vi "TDMS - File Viewer.vi"(4 "error in (no error)":errorcluster, 7 "file path":path) -> (0 "error out":errorcluster, 3 "file path out":path)   [LabVIEW 2020]
doc: "Opens the .tdms file specified in the <B>file in</B> input and presents the file data in the TDMS File Viewer dialog box."
uses:
  <vilib>/Utility/tdmsutil.llb/fileViewerConfigData.ctl
  <vilib>/Utility/error.llb/DialogType.ctl
  <vilib>/event_ctls.llb/sizeaction.ctl
  <vilib>/event_ctls.llb/panelstate.ctl
  <vilib>/Utility/tdmsutil.llb/TDMSFileViewerLocalizedText.vi
  Instance           1 26Saved   TDMS - File Viewer .vi
panel:
  out "LastXScaleFormat":u8
  out "TotalCount":u64
  out "Temp Configuration":T1
  in  "LastTopLeftValue":u64
  out "Resize?":bool
  in  "Help":bool
  in  "Status":string
  in  "Quit":bool
  in  "Settings...":bool
  in  "Properties / Values / Graph":T2(tab)
  in  "Properties":i32(listbox)
  in  "Go To":bool
  in  "Scrollbar":u64(c297)
  in  "Raw data values":i32(listbox)
  out "Waveform Graph":waveform(dbl)[](graph)
  in  "File contents":string(tree)
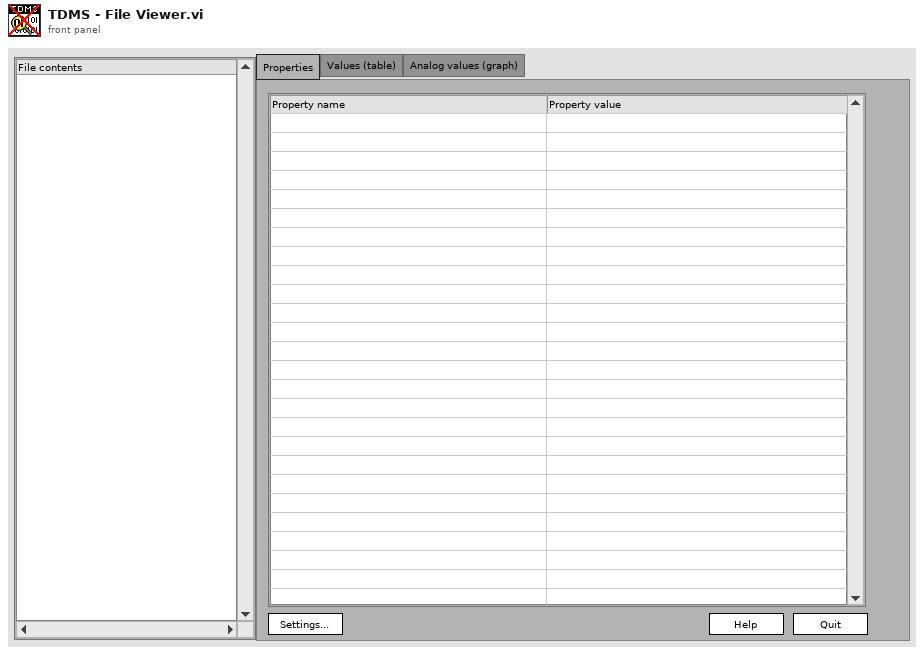
[diagram p1: front panel]
types:
  T1 = typedef "fileViewerConfigData.ctl" = cluster{"Show all (table)":bool, "Show all (graph)":bool, "limit (table)":u64, "limit (graph)":u64, "no show":bool, "start (table)":u64, "start (graph)":u64}
  T2 = enum32{"Properties", "Values (table)", "Analog values (graph)"}
  T3 = enum16{"open", "open or create", "create or replace", "create", "open (read-only)"}
  T4 = cluster{"Tree":refnum<vi>, "Tab Control":refnum<vi>, "property list":refnum<vi>, "raw data list":refnum<vi>, "Waveform Graph":refnum<vi>, "Ok":refnum<vi>, "Ok 2":refnum<vi>, "Ok 3":refnum<vi>, "Ok 4":refnum<vi>, "Scrollbar":refnum<vi>, "Ok 5":refnum<vi>, "TopLeftValue":refnum<vi>, "TotalCount":refnum<vi>}
  T5 = typedef "panelstate.ctl" = enum32{"Standard", "Minimized", "Maximized"}
  T6 = typedef "sizeaction.ctl" = enum32{"Minimized", "Maximized", "Resized"}
  T7 = cluster{"Shift":bool, "Ctrl":bool, "Alt":bool, "Cmd":bool, "Opt":bool}
  T8 = typedef "LVRectTypeDef.ctl" = cluster{"Left":i16, "Top":i16, "Right":i16, "Bottom":i16}
  T9 = typedef "LVRowAndColumnUnsignedTypeDef.ctl" = cluster{"Row":u32, "Column":u32}
  T10 = typedef "DialogType.ctl" = u16
  T11 = typedef "eventvkey.ctl" = enum16{"ASCII", "Enter", "Return", "Shift", "Ctrl", "Alt", "Cmd", "Opt", "Caps", "NumLock", "Clear", "Break", "Up", "Down", "Left", "Right", "Insert", "Delete", "Home", "End", "PageUp", "PageDown", "Escape", "Help", "Pause", "ScrollLock", "F1", "F2", "F3", "F4", "F5", "F6", "F7", "F8", "F9", "F10", "F11", "F12", "F13", "F14", "F15", "F16", "F17", "F18", "F19", "F20", "F21", "F22", "F23", "F24", "Play", "VolumeUp", "VolumeDown", "Mute", "Two Byte Char"}
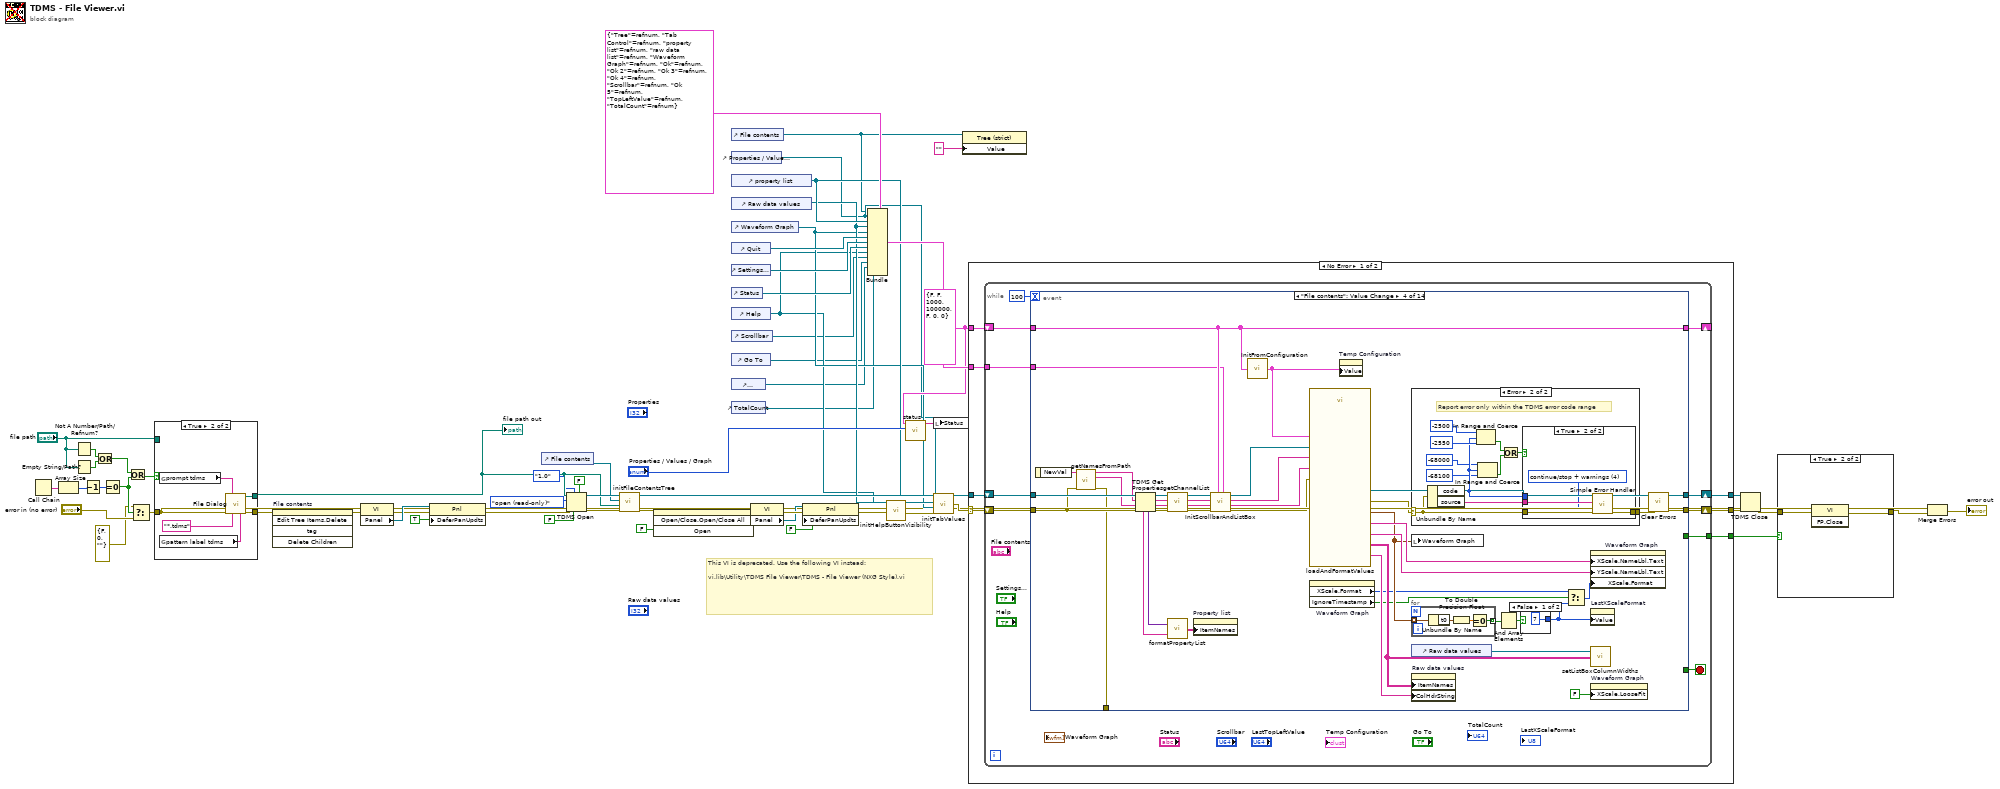
[diagram p0: block diagram]
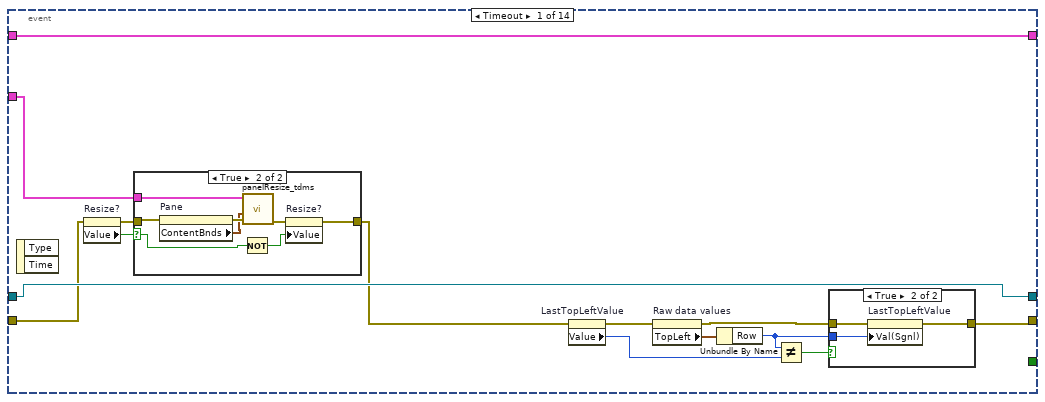
[diagram p3: hidden frame]
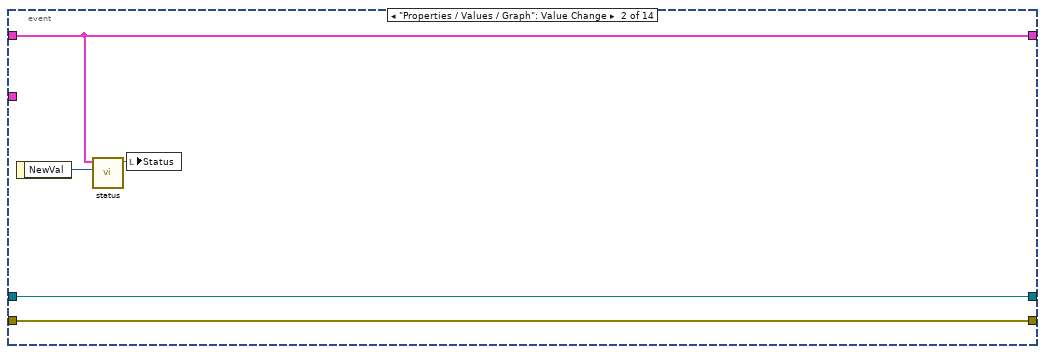
[diagram p6: hidden frame]
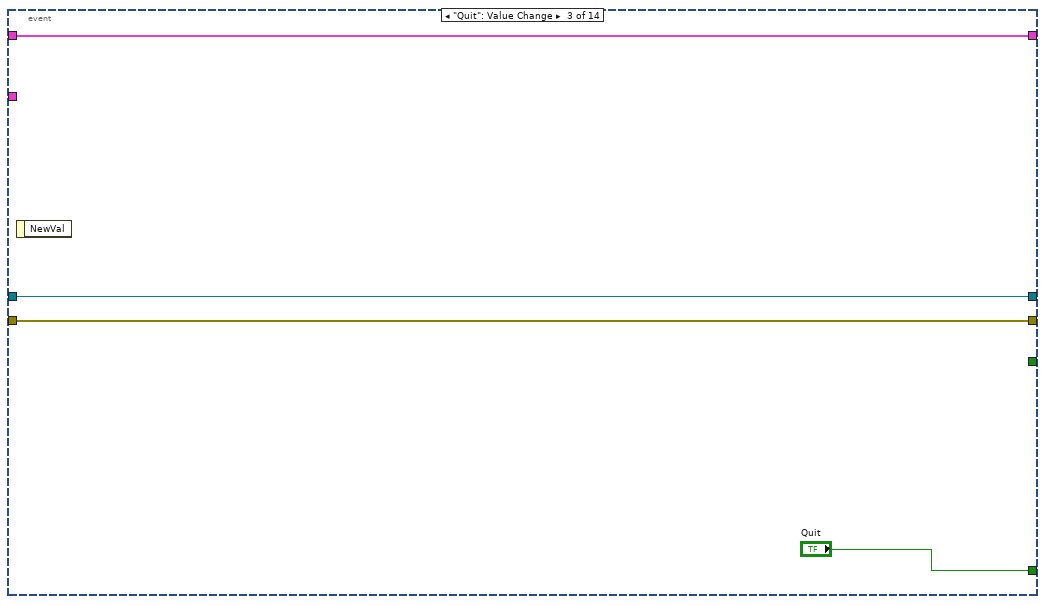
[diagram p7: hidden frame]
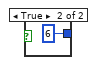
[diagram p8: hidden frame]
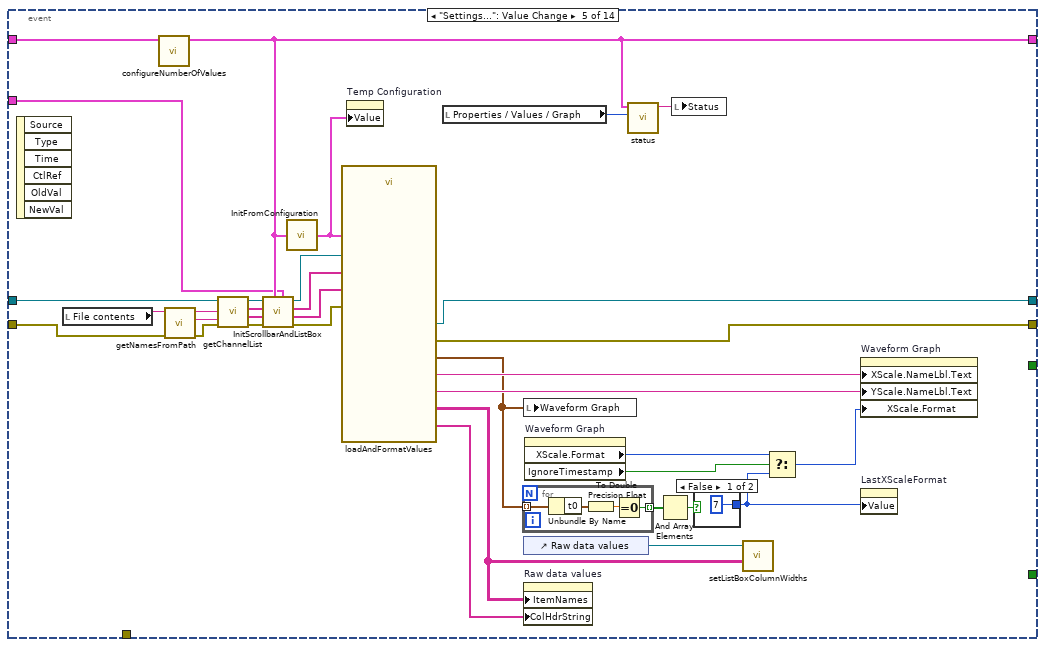
[diagram p11: hidden frame]
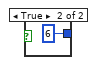
[diagram p12: hidden frame]
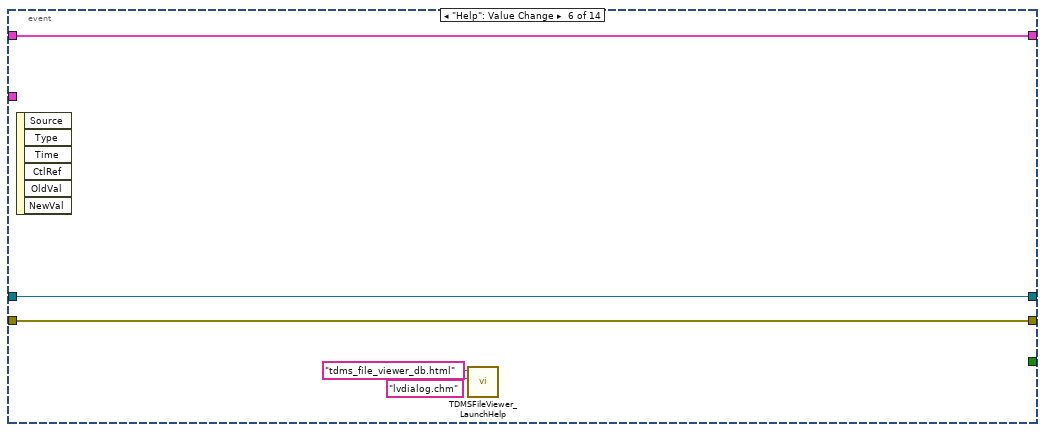
[diagram p13: hidden frame]
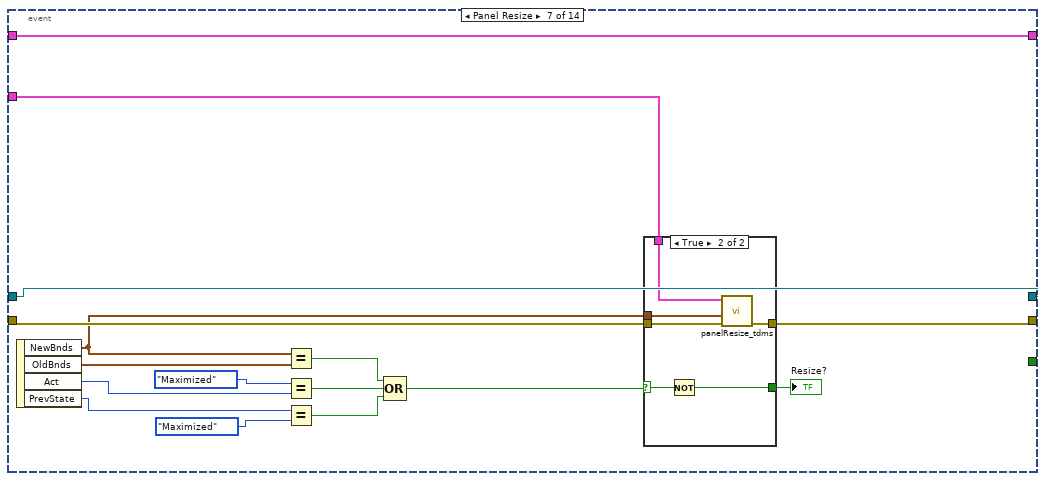
[diagram p14: hidden frame]
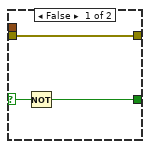
[diagram p15: hidden frame]
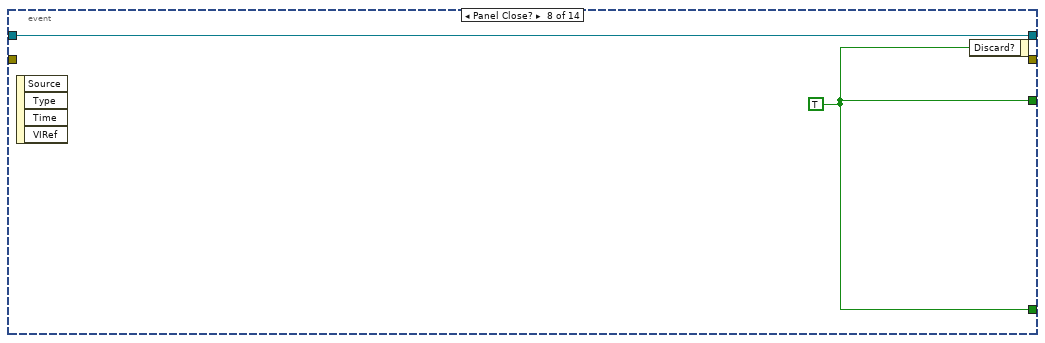
[diagram p16: hidden frame]
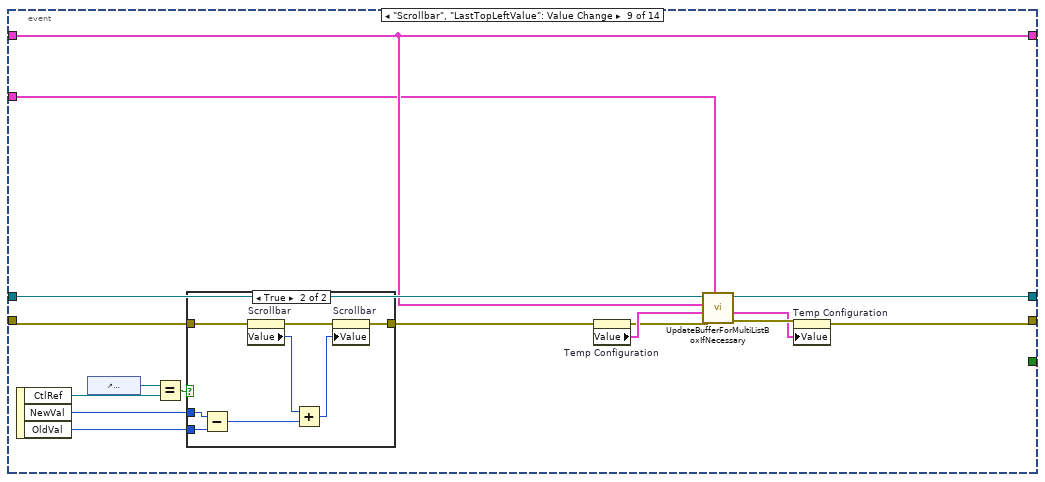
[diagram p17: hidden frame]
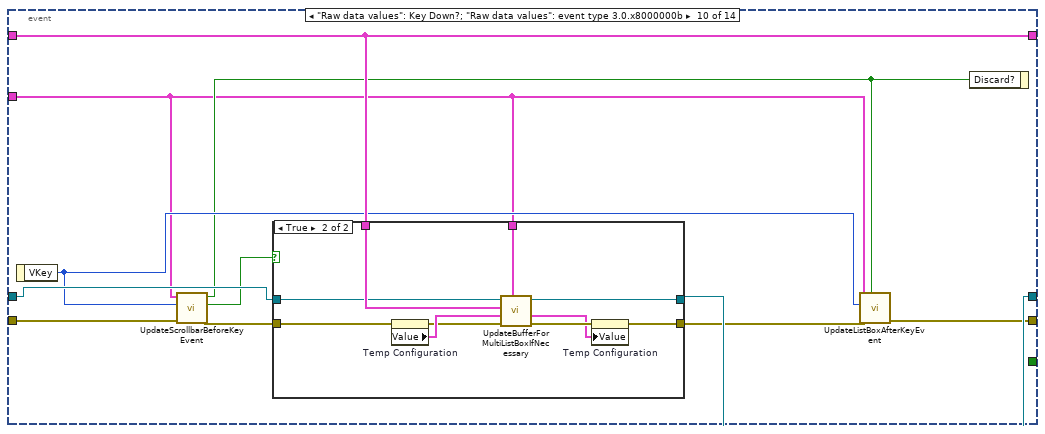
[diagram p19: hidden frame]
diagram:
  w27 = T1 {"Show all (table)"=FALSE, "Show all (graph)"=FALSE, "limit (table)"=1000, "limit (graph)"=100000, "no show"=FALSE, "start (table)"=0, "start (graph)"=0} ("TDMS File Viewer Configuration")
  # "This VI is deprecated. Use the following VI instead:\n\nvi.lib\\Utility\\TDMS File Viewer\\TDMS - File Viewer (NXG Style).vi"
  n1 = Call Chain() -> (call chain=w42:string[])
  n2 = Array Size(array=w42) -> (size(s)=w40:i32)
  n3 = Not A Number/Path/Refnum?(number/path/refnum="file path") -> (NaN/Path/Refnum?=w44:bool)
  n4 = Empty String/Path?(string/path="file path") -> (empty?=w43:bool)
  n5 = Decrement(x=w40) -> (x-1=w39:i32)
  n6 = Or(x=w44, y=w43) -> (x .or. y?=w41:bool)
  n7 = Equal To 0?(x=w39) -> (x = 0?=w25:bool)
  n8 = Or(x=w41, y=w25) -> (x .or. y?=w38:bool)
  n9 = Select(t=errorcluster {"status"=FALSE, "code"=0, "source"=""}, s=w25, f="error in (no error)") -> (s? t:f=w6:errorcluster)
  n10 = case shown="True" w38 {
    tunnel: [w63 w69] -> w31
    tunnel: "file path" -> [w63 _]
    tunnel: [w62 w67] -> w30
    tunnel: w6 -> [w62 w66]
    frame False {
    }
    frame True {
      n11 = global read "TDMSFileViewerLocalizedText.vi" "prompt tdms"() -> (w65:string)
      n12 = global read "TDMSFileViewerLocalizedText.vi" "pattern label tdms"() -> (w64:string)
      n13 = call "File Dialog"("prompt"=w65, "error in"=w66, "pattern (all files)"="*.tdms", "pattern label"=w64) -> ("selected path"=w69:path, "error out"=w67:errorcluster)  [unwired: 3 in, 7 out]
    }
  }
  "file path out" <- w31
  n14 = invoke on="File contents" class="Tree (strict)" method="Edit Tree Items.Delete"(error in=w30) -> (error out=w52:errorcluster)  [unwired: 4 in, 4 out]
  n15 = property class="VI"(error in=w52) -> (error out=w53:errorcluster, "Panel"=w54:refnum<vi>)  [unwired: 1 in, 1 out]
  n16 = property class="Pnl"(reference=w54, error in=w53, "DeferPanUpdts"=TRUE ("Defer Panel Updates")) -> (error out=w56:errorcluster)  [unwired: 1 out]
  n17 = control-ref of="File contents"() -> (w32:refnum<vi>)
  n18 = TDMS Open(5:FALSE ("create index file? (T)"), 6:FALSE ("disable buffering (T)"), 7:enum16{"1.0", "2.0"}."1.0" ("file format version (2.0)"), 8:w56, 10:T3."open (read-only)" ("operation"), 11:w31) -> (0:w61:errorcluster, 3:w60:refnum<k34>)  [unwired: 1 in]
  n19 = call <vilib>:"initFileContentsTree.vi"("error in (no error)"=w61, "file path"=w31, "Tree Refnum"=w32, "tdms file"=w60) -> ("error out"=w48:errorcluster, "tdms file out"=w59:refnum<k34>)  [unwired: 2 out]
  n20 = invoke on="File contents" class="Tree (strict)" method="Open/Close.Open/Close All"(error in=w48, "Open"=FALSE ("Open?")) -> (error out=w47:errorcluster)  [unwired: 2 in, 3 out]
  n21 = control-ref of="File contents"() -> (w13:refnum<vi>)
  n22 = control-ref of="Properties / Values / Graph"() -> (w14:refnum<vi>)
  n23 = control-ref of="property list"() -> (w17:refnum<vi>)
  n24 = control-ref of="Raw data values"() -> (w16:refnum<vi>)
  n25 = control-ref of="Waveform Graph"() -> (w15:refnum<vi>)
  n26 = control-ref of="Quit"() -> (w36:refnum<vi>)
  n27 = control-ref of="Settings..."() -> (w34:refnum<vi>)
  n28 = control-ref of="Status"() -> (w29:refnum<vi>)
  n29 = control-ref of="Help"() -> (w9:refnum<vi>)
  n30 = control-ref of="Scrollbar"() -> (w5:refnum<vi>)
  n31 = control-ref of="Go To"() -> (w4:refnum<vi>)
  n32 = control-ref of="LastTopLeftValue"() -> (w3:refnum<vi>)
  n33 = control-ref of="TotalCount"() -> (w2:refnum<vi>)
  n34 = property class="VI"(error in=w47) -> (error out=w50:errorcluster, "Panel"=w49:refnum<vi>)  [unwired: 1 in, 1 out]
  n35 = property class="Pnl"(reference=w49, error in=w50, "DeferPanUpdts"=FALSE ("Defer Panel Updates")) -> (error out=w11:errorcluster)  [unwired: 1 out]
  n36 = Bundle(cluster=T4 {"Tree"=refnum, "Tab Control"=refnum, "property list"=refnum, "raw data list"=refnum, "Waveform Graph"=refnum, "Ok"=refnum, "Ok 2"=refnum, "Ok 3"=refnum, "Ok 4"=refnum, "Scrollbar"=refnum, "Ok 5"=refnum, "TopLeftValue"=refnum, "TotalCount"=refnum} ("control refs"), "Tree"=w13, "Tab Control"=w14, "property list"=w17, "raw data list"=w16, "Waveform Graph"=w15, "Ok"=w36, "Ok 2"=w34, "Ok 3"=w29, "Ok 4"=w9, "Scrollbar"=w5, "Ok 5"=w4, "TopLeftValue"=w3, "TotalCount"=w2) -> (w37:T4)
  n37 = call <vilib>:"initHelpButtonVisibility.vi"("error in"=w11, "Help"=w9) -> ("error out"=w10:errorcluster)  [unwired: 9 in]
  n38 = call <vilib>:"status.vi"("tab sheet"="Properties / Values / Graph", "TDMS File Viewer Configuration"=w27) -> ("status"=w28:string)  [unwired: 5 out]
  n39 = local write "Status"(w28) -> ()
  n40 = call <vilib>:"initTabValues.vi"("properties"=w17, "Values"=w16, "waveform"=w15, "error in"=w10, "Properties / Values / Graph"=w14) -> ("error out"=w18:errorcluster)
  n41 = property class="Tree (strict)"(reference=w13, "Value"="") -> ()  [unwired: 1 in, 2 out]
  n42 = case shown="No Error" w18 {
    selector: w18 -> [w71 w393]
    tunnel: w59 -> [w76 w394]
    tunnel: [w75 w394] -> w58
    tunnel: [w74 w392] -> w57
    tunnel: w37 -> [w73 _]
    tunnel: w27 -> [w72 _]
    tunnel: [w70 FALSE] -> w22
    frame No Error {
      n43 = while {
        shift-right: [w84] -> w74
        shift-left: w71 -> [w85]
        shift-right: [w83] -> w75
        shift-left: w76 -> [w86]
        tunnel: w73 -> [w81]
        shift-right: [w79] -> _
        shift-left: w72 -> [w80]
        tunnel: [w78] -> w70
        stop <- w82 stop-if-true
        n44 = event shown="[3] \"File contents\": Value Change" {
          selector: _ -> [_ _ _ _ _ _ _ _ _ _ _ _ _ _]
          dyn-events: _ -> [_ _ _ _ _ _ _ _ _ _ _ _ _ _]
          timeout: 100 -> [_ _ _ _ _ _ _ _ _ _ _ _ _ _]
          tunnel: w86 -> [w100 w117 w121 w163 w211 w231 w248 w259 w275 w294 w319 w334 w367 w384]
          tunnel: w85 -> [w95 w118 w120 w155 w218 w230 w246 _ w262 w286 w308 w331 w366 w383]
          tunnel: [w88 w118 w120 w151 w219 w230 w245 _ w269 w291 w311 w332 w366 w375] -> w84
          tunnel: [w100 w117 w121 w162 w220 w231 w248 w259 w274 w293 w318 w333 w367 w384] -> w83
          tunnel: [_ _ "Quit" _ _ _ _ w258 _ _ _ _ _ _] -> w82
          tunnel: [_ _ _ w154 _ _ _ _ _ _ _ _ _ _] -> _
          tunnel: w81 -> [w96 _ _ w130 w195 _ w247 _ w261 w287 w309 w328 _ _]
          tunnel: w80 -> [w99 w114 w119 w131 w221 w232 w244 _ w273 w295 w320 w335 w368 w385]
          tunnel: [w99 w114 w119 w131 w197 w232 w244 _ w273 w295 w320 w335 w368 w385] -> w79
          tunnel: [_ _ _ _ _ _ _ w258 _ _ _ _ _ _] -> w78
          event Timeout {
            n45 = event-data() -> ()  [unwired: 3 out]
            n46 = property on="Resize?" class="Bool (strict)"(error in=w95) -> (error out=w97:errorcluster, "Value"=w98:bool)  [unwired: 1 in, 1 out]
            n47 = case shown="True" w98 {
              selector: w98 -> [_ w112]
              tunnel: w96 -> [_ w113]
              tunnel: w97 -> [w105 w108]
              tunnel: [w105 w110] -> w93
              frame False {
              }
              frame True {
                n48 = property on="Pane" class="Pane"(error in=w108) -> (error out=w107:errorcluster, "ContentBnds"=w106:T8)  [unwired: 1 in, 1 out]
                n49 = Not(x=w112) -> (.not. x?=w109:bool)
                n50 = call <vilib>:"panelResize_tdms.vi"("error in (no error)"=w107, "NewBnds"=w106, "control refs"=w113) -> ("error out"=w111:errorcluster)  [unwired: 4 in]
                n51 = property on="Resize?" class="Bool (strict)"(error in=w111, "Value"=w109) -> (error out=w110:errorcluster)  [unwired: 1 in, 1 out]
              }
            }
            n52 = property on="LastTopLeftValue" class="DigNum (strict)"(error in=w93) -> (error out=w92:errorcluster, "Value"=w91:u64)  [unwired: 1 in, 1 out]
            n53 = property on="Raw data values" class="MCListbox (strict)"(error in=w92) -> (error out=w89:errorcluster, "TopLeft"=w94:T9)  [unwired: 1 in, 1 out]
            n54 = Unbundle By Name(w94) -> ("Row"=w87:u32)
            n55 = Not Equal?(x=w87, y=w91) -> (x != y?=w90:bool)
            n56 = case shown="True" w90 {
              tunnel: w89 -> [w101 w104]
              tunnel: [w101 w103] -> w88
              tunnel: w87 -> [_ w102]
              frame False {
              }
              frame True {
                n57 = property on="LastTopLeftValue" class="DigNum (strict)"(error in=w104, "Val(Sgnl)"=w102) -> (error out=w103:errorcluster)  [unwired: 1 in, 1 out]
              }
            }
          }
          event "Properties / Values / Graph": Value Change {
            n58 = event-data() -> ("NewVal"=w116:T2)  [unwired: 1 out]
            n59 = call <vilib>:"status.vi"("tab sheet"=w116, "TDMS File Viewer Configuration"=w114) -> ("status"=w115:string)  [unwired: 5 out]
            n60 = local write "Status"(w115) -> ()
          }
          event "Quit": Value Change {
            n61 = event-data() -> ()  [unwired: 2 out]
          }
          event "File contents": Value Change {
            n62 = event-data() -> ("NewVal"=w157:string)  [unwired: 1 out]
            n63 = call <vilib>:"getNamesFromPath.vi"("error in (no error)"=w155, "tree path"=w157) -> ("error out"=w154:errorcluster, "channel"=w160:string, "group"=w161:string)  [unwired: 3 out]
            n64 = TDMS Get Properties(8:w155, 9:w160, 10:w161, 11:w163) -> (0:w149:errorcluster, 1:w148:string, 2:w144:string, 3:w150:refnum<k34>, 4:w158:variant[], 6:w159:string[])  [unwired: 2 out]
            n65 = call <vilib>:"getChannelList.vi"("error in (no error)"=w149, "channel names"=w148, "group name"=w144, "tdms file"=w150) -> ("error out"=w139:errorcluster, "channel names out"=w137:string[], "group names out"=w135:string[], "tdms file out"=w133:refnum<k34>)
            n66 = call <vilib>:"formatPropertyList.vi"("property names"=w159, "property values"=w158) -> ("strings"=w156:string[][])
            n67 = property on="Property list" class="MCListbox (strict)"("ItemNames"=w156) -> ()  [unwired: 2 in, 2 out]
            n68 = call <vilib>:"InitScrollbarAndListBox.vi"("control refs"=w130, "configuration"=w131, "error in (no error)"=w139, "channel names"=w137, "group names"=w135, "tdms in"=w133) -> ("error out"=w138:errorcluster, "channel out"=w136:string[], "group out"=w134:string[], "tdms out"=w132:refnum<k34>)  [unwired: 2 in]
            n69 = call <vilib>:"InitFromConfiguration.vi"("configuration"=w131) -> ("output cluster"=w140:T1)  [unwired: 4 in]
            n70 = call <vilib>:"loadAndFormatValues.vi"("error in (no error)"=w138, "configuration"=w140, "channel names"=w136, "group names"=w134, "tdms file"=w132) -> ("error out"=w143:errorcluster, "graph y names"=w146:string, "graph x names"=w145:string, "tdms file out"=w162:refnum<k34>, "waveform values"=w129:waveform(dbl)[], "table values"=w153:string[][], "table headers"=w147:string[])
            n71 = property on="Waveform Graph" class="WFGraph (strict)"() -> ("XScale.Format"=w124:u8, "IgnoreTimestamp"=w123:bool)  [unwired: 2 in, 2 out]
            n72 = property on="Temp Configuration" class="Clust (strict)"("Value"=w140) -> ()  [unwired: 2 in, 2 out]
            n73 = case shown="Error" w143 {
              selector: w143 -> [w170 w180]
              tunnel: [w170 w179] -> w142
              frame No Error {
              }
              frame Error {
                # "Report error only within the TDMS error code range"
                n74 = Unbundle By Name(w180) -> ("code"=w176:i32, "source"=w181:string)
                n75 = In Range and Coerce(upper limit=-2500, x=w176, lower limit=-2550 ("upper limit")) -> (In Range?=w173:bool)  [unwired: 1 out]
                n76 = In Range and Coerce(upper limit=-68000, x=w176, lower limit=-68100) -> (In Range?=w172:bool)  [unwired: 1 out]
                n77 = Or(x=w173, y=w172) -> (x .or. y?=w171:bool)
                n78 = case shown="True" w171 {
                  tunnel: w181 -> [_ w187]
                  tunnel: w180 -> [w182 w186]
                  tunnel: [w182 w185] -> w179
                  tunnel: w176 -> [_ w183]
                  frame False {
                    # "Out of the range of TDMS\nerror code, we don't report\nthem."
                  }
                  frame True {
                    w184 = T10 4 items=["no dialog", "OK message", "continue or stop message", "OK message + warnings", "continue/stop + warnings"] ("type of dialog (OK msg:1)")
                    n79 = call <vilib>:"Simple Error Handler.vi"("error code (no error:0)"=w183, "error source (\" \")"=w187, "type of dialog (OK msg:1)"=w184, "error in (no error)"=w186) -> ("error out"=w185:errorcluster)  [unwired: 1 in, 4 out]
                  }
                }
              }
            }
            n80 = local write "Waveform Graph"(w129) -> ()
            n81 = for {
              tunnel: w129 -> [w169] mode=indexing
              tunnel: [w166] -> w128 mode=indexing
              n82 = Unbundle By Name(w169) -> ("t0"=w168:timestamp)
              n83 = To Double Precision Float(number=w168) -> (double precision float=w167:dbl)
              n84 = Equal To 0?(x=w167) -> (x = 0?=w166:bool)
            }
            n85 = control-ref of="Raw data values"() -> (w152:refnum<vi>)
            n86 = property on="Raw data values" class="MCListbox (strict)"("ItemNames"=w153, "ColHdrString"=w147) -> ()  [unwired: 2 in, 2 out]
            n87 = And Array Elements(Boolean array=w128) -> (logical AND=w127:bool)
            n88 = case shown="False" w127 {
              tunnel: [u8 7 u8 6] -> w125
              frame False {
              }
              frame True {
              }
            }
            n89 = Select(t=w124, s=w123, f=w125) -> (s? t:f=w126:u8)
            n90 = property on="Waveform Graph" class="WFGraph (strict)"("XScale.NameLbl.Text"=w145, "YScale.NameLbl.Text"=w146, "XScale.Format"=w126) -> ()  [unwired: 2 in, 2 out]
            n91 = property on="LastXScaleFormat" class="DigNum (strict)"("Value"=w125) -> ()  [unwired: 2 in, 2 out]
            n92 = call <vilib>:"setListBoxColumnWidths.vi"("table data"=w153, "MCListbox Refnum"=w152) -> ()  [unwired: 1 out]
            n93 = property on="Waveform Graph" class="WFGraph (strict)"("XScale.LooseFit"=FALSE ("X Scale.Loose Fit")) -> ()  [unwired: 2 in, 2 out]
            n94 = call <vilib>:"Clear Errors.vi"("error in (no error)"=w142) -> ("error out"=w151:errorcluster)  [unwired: 1 in, 5 out]
          }
          event "Settings...": Value Change {
            n95 = event-data() -> ()  [unwired: 7 out]
            n96 = local read "File contents"() -> (w212:string)
            n97 = call <vilib>:"configureNumberOfValues.vi"("TDMS File Viewer Configuration"=w221) -> ("TDMS File Viewer Configuration Out"=w197:T1)  [unwired: 10 out]
            n98 = call <vilib>:"getNamesFromPath.vi"("error in (no error)"=w218, "tree path"=w212) -> ("error out"=w210:errorcluster, "channel"=w208:string, "group"=w209:string)  [unwired: 3 out]
            n99 = call <vilib>:"getChannelList.vi"("error in (no error)"=w210, "channel names"=w208, "group name"=w209, "tdms file"=w211) -> ("error out"=w199:errorcluster, "channel names out"=w201:string[], "group names out"=w203:string[], "tdms file out"=w205:refnum<k34>)
            n100 = call <vilib>:"InitScrollbarAndListBox.vi"("control refs"=w195, "configuration"=w197, "error in (no error)"=w199, "channel names"=w201, "group names"=w203, "tdms in"=w205) -> ("error out"=w198:errorcluster, "channel out"=w200:string[], "group out"=w202:string[], "tdms out"=w204:refnum<k34>)  [unwired: 2 in]
            n101 = call <vilib>:"InitFromConfiguration.vi"("configuration"=w197) -> ("output cluster"=w196:T1)  [unwired: 4 in]
            n102 = call <vilib>:"loadAndFormatValues.vi"("error in (no error)"=w198, "configuration"=w196, "channel names"=w200, "group names"=w202, "tdms file"=w204) -> ("error out"=w219:errorcluster, "graph y names"=w214:string, "graph x names"=w213:string, "tdms file out"=w220:refnum<k34>, "waveform values"=w192:waveform(dbl)[], "table values"=w215:string[][], "table headers"=w217:string[])
            n103 = property on="Temp Configuration" class="Clust (strict)"("Value"=w196) -> ()  [unwired: 2 in, 2 out]
            n104 = local read "Properties / Values / Graph"() -> (w206:T2)
            n105 = for {
              tunnel: w192 -> [w227] mode=indexing
              tunnel: [w224] -> w194 mode=indexing
              n106 = Unbundle By Name(w227) -> ("t0"=w226:timestamp)
              n107 = To Double Precision Float(number=w226) -> (double precision float=w225:dbl)
              n108 = Equal To 0?(x=w225) -> (x = 0?=w224:bool)
            }
            n109 = local write "Waveform Graph"(w192) -> ()
            n110 = control-ref of="Raw data values"() -> (w216:refnum<vi>)
            n111 = property on="Raw data values" class="MCListbox (strict)"("ItemNames"=w215, "ColHdrString"=w217) -> ()  [unwired: 2 in, 2 out]
            n112 = property on="Waveform Graph" class="WFGraph (strict)"() -> ("XScale.Format"=w189:u8, "IgnoreTimestamp"=w188:bool)  [unwired: 2 in, 2 out]
            n113 = call <vilib>:"status.vi"("tab sheet"=w206, "TDMS File Viewer Configuration"=w197) -> ("status"=w207:string)  [unwired: 5 out]
            n114 = And Array Elements(Boolean array=w194) -> (logical AND=w193:bool)
            n115 = local write "Status"(w207) -> ()
            n116 = case shown="False" w193 {
              tunnel: [u8 7 u8 6] -> w190
              frame False {
              }
              frame True {
              }
            }
            n117 = call <vilib>:"setListBoxColumnWidths.vi"("table data"=w215, "MCListbox Refnum"=w216) -> ()  [unwired: 1 out]
            n118 = Select(t=w189, s=w188, f=w190) -> (s? t:f=w191:u8)
            n119 = property on="Waveform Graph" class="WFGraph (strict)"("XScale.NameLbl.Text"=w213, "YScale.NameLbl.Text"=w214, "XScale.Format"=w191) -> ()  [unwired: 2 in, 2 out]
            n120 = property on="LastXScaleFormat" class="DigNum (strict)"("Value"=w190) -> ()  [unwired: 2 in, 2 out]
          }
          event "Help": Value Change {
            n121 = event-data() -> ()  [unwired: 7 out]
            n122 = call <vilib>:"TDMSFileViewer_LaunchHelp.vi"("CHM or HLP filename (lvdialog.chm)"="lvdialog.chm", "HTML filename"="tdms_file_viewer_db.html") -> ()  [unwired: 1 in, 5 out]
          }
          event Panel Resize {
            n123 = event-data() -> ("NewBnds"=w236:T8, "OldBnds"=w235:T8, "Act"=w237:T6, "PrevState"=w238:T5)  [unwired: 1 out]
            n124 = Equal?(x=w236, y=w235) -> (x = y?=w241:bool)
            n125 = Equal?(x=sizeaction."Maximized" ("Act"), y=w237) -> (x = y?=w240:bool)
            n126 = Equal?(x=w238, y=panelstate."Maximized" ("PrevState")) -> (x = y?=w239:bool)
            n127 = Compound Arithmetic op=OR(w241, w240, w239) -> (w234:bool)
            n128 = case shown="True" w234 {
              selector: w234 -> [w250 w253]
              tunnel: w247 -> [_ w257]
              tunnel: w246 -> [w251 w256]
              tunnel: [w251 w255] -> w245
              tunnel: w236 -> [_ w254]
              tunnel: [w249 w252] -> w233
              frame False {
                n129 = Not(x=w250) -> (.not. x?=w249:bool)
              }
              frame True {
                n130 = Not(x=w253) -> (.not. x?=w252:bool)
                n131 = call <vilib>:"panelResize_tdms.vi"("error in (no error)"=w256, "NewBnds"=w254, "control refs"=w257) -> ("error out"=w255:errorcluster)  [unwired: 4 in]
              }
            }
            "Resize?" <- w233
          }
          event Panel Close? {
            w258 = TRUE
            n132 = event-data() -> ()  [unwired: 5 out]
            n133 = event-data("Discard?"=w258) -> ()  [unwired: 1 in, 1 out]
          }
          event "Scrollbar", "LastTopLeftValue": Value Change {
            n134 = event-data() -> ("CtlRef"=w267:refnum<vi>, "NewVal"=w264:u64, "OldVal"=w263:u64)  [unwired: 1 out]
            n135 = control-ref of="LastTopLeftValue"() -> (w266:refnum<vi>)
            n136 = Equal?(x=w266, y=w267) -> (x = y?=w265:bool)
            n137 = case shown="True" w265 {
              tunnel: w264 -> [_ w280]
              tunnel: w263 -> [_ w279]
              tunnel: w262 -> [w276 w278]
              tunnel: [w276 w277] -> w260
              frame False {
              }
              frame True {
                n138 = Subtract(x=w280, y=w279) -> (x-y=w282:u64)
                n139 = property on="Scrollbar" class="Scroll (strict)"(error in=w278) -> (error out=w284:errorcluster, "Value"=w283:u64)  [unwired: 1 in, 1 out]
                n140 = Add(x=w283, y=w282) -> (x+y=w281:u64)
                n141 = property on="Scrollbar" class="Scroll (strict)"(error in=w284, "Value"=w281) -> (error out=w277:errorcluster)  [unwired: 1 in, 1 out]
              }
            }
            n142 = property on="Temp Configuration" class="Clust (strict)"(error in=w260) -> (error out=w271:errorcluster, "Value"=w272:T1)  [unwired: 1 in, 1 out]
            n143 = call <vilib>:"UpdateBufferForMultiListBoxIfNecessary.vi"("control refs"=w261, "error in"=w271, "Buffer Configuration"=w272, "TDMS File Viewer Configuration"=w273, "tdms file in"=w275) -> ("error out"=w270:errorcluster, "BufferConfig out"=w268:T1, "tdms file out"=w274:refnum<k34>)  [unwired: 4 in]
            n144 = property on="Temp Configuration" class="Clust (strict)"(error in=w270, "Value"=w268) -> (error out=w269:errorcluster)  [unwired: 1 in, 1 out]
          }
          event "Raw data values": Key Down?; "Raw data values": event type 3.0.x8000000b {
            n145 = event-data() -> ("VKey"=w289:T11)  [unwired: 1 out]
            n146 = call <vilib>:"UpdateScrollbarBeforeKeyEvent.vi"("error in (no error)"=w286, "VKey"=w289, "control refs 2"=w287) -> ("error out"=w292:errorcluster, "LoadBuffer?"=w290:bool, "DiscardEvent?"=w288:bool)  [unwired: 6 in]
            n147 = case shown="True" w290 {
              tunnel: w295 -> [_ w303]
              tunnel: w294 -> [w296 w302]
              tunnel: [w296 w301] -> w293
              tunnel: w292 -> [w297 w298]
              tunnel: [w297 w300] -> w285
              tunnel: w287 -> [_ w299]
              frame False {
              }
              frame True {
                n148 = property on="Temp Configuration" class="Clust (strict)"(error in=w298) -> (error out=w306:errorcluster, "Value"=w307:T1)  [unwired: 1 in, 1 out]
                n149 = call <vilib>:"UpdateBufferForMultiListBoxIfNecessary.vi"("control refs"=w299, "error in"=w306, "Buffer Configuration"=w307, "TDMS File Viewer Configuration"=w303, "tdms file in"=w302) -> ("error out"=w305:errorcluster, "BufferConfig out"=w304:T1, "tdms file out"=w301:refnum<k34>)  [unwired: 4 in]
                n150 = property on="Temp Configuration" class="Clust (strict)"(error in=w305, "Value"=w304) -> (error out=w300:errorcluster)  [unwired: 1 in, 1 out]
              }
            }
            n151 = call <vilib>:"UpdateListBoxAfterKeyEvent.vi"("DiscardEvent?"=w288, "error in (no error)"=w285, "VKey"=w289, "control refs"=w287) -> ("error out"=w291:errorcluster)  [unwired: 7 in]
            n152 = event-data("Discard?"=w288) -> ()  [unwired: 1 in, 1 out]
          }
          event "Go To": Value Change {
            n153 = event-data() -> ()  [unwired: 2 out]
            n154 = call <vilib>:"GoTo.vi"("error in"=w308, "control refs"=w309) -> ("error out"=w317:errorcluster, "VisibleValue"=w314:u64)  [unwired: 8 in]
            n155 = property on="Temp Configuration" class="Clust (strict)"(error in=w317) -> (error out=w323:errorcluster, "Value"=w324:T1)  [unwired: 1 in, 1 out]
            n156 = call <vilib>:"UpdateBufferForMultiListBoxIfNecessary.vi"("control refs"=w309, "error in"=w323, "Buffer Configuration"=w324, "TDMS File Viewer Configuration"=w320, "tdms file in"=w319) -> ("error out"=w322:errorcluster, "BufferConfig out"=w321:T1, "tdms file out"=w318:refnum<k34>)  [unwired: 4 in]
            n157 = property on="Temp Configuration" class="Clust (strict)"(error in=w322, "Value"=w321) -> (error out=w310:errorcluster)  [unwired: 1 in, 1 out]
            n158 = property on="Raw data values" class="MCListbox (strict)"(error in=w310) -> (error out=w312:errorcluster, "TopLeft"=w316:T9)  [unwired: 1 in, 1 out]
            n159 = Unbundle By Name(w316) -> ("Row"=w315:u32)
            n160 = Add(x=w315, y=w314) -> (x+y=w313:u64)
            n161 = property on="Raw data values" class="MCListbox (strict)"(error in=w312, "Value"=w313) -> (error out=w311:errorcluster)  [unwired: 1 in, 1 out]
          }
          event Key Down {
            n162 = event-data() -> ("PlatMods"=w327:T7, "Char"=w326:i16)  [unwired: 1 out]
            n163 = property on="Raw data values" class="MCListbox (strict)"(error in=w331) -> (error out=w325:errorcluster, "Key Focus"=w330:bool)  [unwired: 1 in, 1 out]
            n164 = case shown="True" w330 {
              selector: w330 -> [w336 _]
              tunnel: [w336 w337] -> w329
              tunnel: w327 -> [_ w342]
              tunnel: w326 -> [_ w341]
              frame False {
              }
              frame True {
                n165 = disable-structure shown="Default" {
                  disable-tunnel: [T7 {"Shift"=FALSE, "Ctrl"=TRUE, "Alt"=FALSE, "Cmd"=FALSE, "Opt"=TRUE} ("PlatMods") T7 {"Shift"=FALSE, "Ctrl"=FALSE, "Alt"=FALSE, "Cmd"=TRUE, "Opt"=FALSE} ("PlatMods")] -> w343
                  frame condition #0 (active) {
                  }
                  frame condition #1 {
                  }
                }
                n166 = Equal?(x=w343, y=w342) -> (x = y?=w339:bool)
                n167 = Equal?(x=w341, y=i16 103 ("Char")) -> (x = y?=w338:bool)
                n168 = And(x=w339, y=w338) -> (x .and. y?=w337:bool)
              }
            }
            n169 = case shown="True" w329 {
              tunnel: w335 -> [_ w361]
              tunnel: w334 -> [w346 w360]
              tunnel: [w346 w359] -> w333
              tunnel: [w347 w352] -> w332
              tunnel: w325 -> [w347 w348]
              tunnel: w328 -> [_ w350]
              tunnel: w328 -> [_ w349]
              frame False {
              }
              frame True {
                n170 = call <vilib>:"GoTo.vi"("error in"=w348, "control refs"=w349) -> ("error out"=w358:errorcluster, "VisibleValue"=w355:u64)  [unwired: 8 in]
                n171 = property on="Temp Configuration" class="Clust (strict)"(error in=w358) -> (error out=w364:errorcluster, "Value"=w365:T1)  [unwired: 1 in, 1 out]
                n172 = call <vilib>:"UpdateBufferForMultiListBoxIfNecessary.vi"("control refs"=w350, "error in"=w364, "Buffer Configuration"=w365, "TDMS File Viewer Configuration"=w361, "tdms file in"=w360) -> ("error out"=w363:errorcluster, "BufferConfig out"=w362:T1, "tdms file out"=w359:refnum<k34>)  [unwired: 4 in]
                n173 = property on="Temp Configuration" class="Clust (strict)"(error in=w363, "Value"=w362) -> (error out=w351:errorcluster)  [unwired: 1 in, 1 out]
                n174 = property on="Raw data values" class="MCListbox (strict)"(error in=w351) -> (error out=w353:errorcluster, "TopLeft"=w357:T9)  [unwired: 1 in, 1 out]
                n175 = Unbundle By Name(w357) -> ("Row"=w356:u32)
                n176 = Add(x=w356, y=w355) -> (x+y=w354:u64)
                n177 = property on="Raw data values" class="MCListbox (strict)"(error in=w353, "Value"=w354) -> (error out=w352:errorcluster)  [unwired: 1 in, 1 out]
              }
            }
          }
          event Key Down? {
            n178 = event-data() -> ("VKey"=w370:T11)  [unwired: 1 out]
            n179 = case shown="\"F1\"" w370 {
              tunnel: [FALSE ("Discard?") TRUE ("Discard?")] -> w369
              frame Default {
              }
              frame "F1" {
                n180 = call <vilib>:"TDMSFileViewer_LaunchHelp.vi"("CHM or HLP filename (lvdialog.chm)"="lvdialog.chm", "HTML filename"="tdms_file_viewer_db.html") -> ()  [unwired: 1 in, 5 out]
              }
            }
            n181 = event-data("Discard?"=w369) -> ()  [unwired: 1 in, 1 out]
          }
          event "Waveform Graph": Shortcut Menu Selection (App) {
            n182 = event-data() -> ("ItemTag"=w381:string)  [unwired: 1 out]
            n183 = property on="Waveform Graph" class="WFGraph (strict)"(error in=w383) -> (error out=w376:errorcluster, "IgnoreTimestamp"=w380:bool)  [unwired: 1 in, 1 out]
            n184 = Not(x=w380) -> (.not. x?=w377:bool)
            n185 = Equal?(x=w381, y="APP_SC_IGNORE_TIME_STAMP") -> (x = y?=w378:bool)
            n186 = And(x=w377, y=w378) -> (x .and. y?=w379:bool)
            n187 = case shown="True" w379 {
              tunnel: w376 -> [w386 w390]
              tunnel: [w386 w387] -> w375
              frame False {
              }
              frame True {
                n188 = property on="LastXScaleFormat" class="DigNum (strict)"(error in=w390) -> (error out=w389:errorcluster, "Value"=w388:u8)  [unwired: 1 in, 1 out]
                n189 = property on="Waveform Graph" class="WFGraph (strict)"(error in=w389, "XScale.Format"=w388) -> (error out=w387:errorcluster)  [unwired: 1 in, 1 out]
              }
            }
          }
        }
      }
    }
    frame Error {
      n190 = call <vilib>:"Simple Error Handler.vi"("error in (no error)"=w393) -> ("error out"=w392:errorcluster)  [unwired: 1 in, 7 out]
    }
  }
  n191 = TDMS Close(8:w57, 11:w58) -> (0:w21:errorcluster)  [unwired: 1 out]
  n192 = case shown="True" w22 {
    tunnel: w21 -> [w395 w397]
    tunnel: [w395 w396] -> w8
    frame False {
    }
    frame True {
      n193 = invoke class="VI" method="FP.Close"(error in=w397) -> (error out=w396:errorcluster)  [unwired: 2 in, 2 out]
    }
  }
  n194 = Merge Errors(w6, w8) -> (→"error out":errorcluster)
